vi "Node - Read Local Table.vi"(8 "error in (no error)":errorcluster, 10 "Node Name":string, 11 "Compiled.Settings In":T1) -> (0 "error out":errorcluster, 2 "Local Channels Table out":string[][](array[string]), 3 "Compiled.Settings Out":T1)   [LabVIEW 2016, in "PXImc Custom Device System Explorer.lvlib"]
uses:
  PXImc Custom Device System Explorer.lvlib
  Shared/Compiled.Settings.ctl
  <vilib>/NI Veristand/VeriStand Data/Byte Buffer/Byte Buffer.lvclass
  PXImc Router/Controls/Target Type.ctl
  PXImc Router/Controls/Router - Configuration.ctl
  PXImc Router/Controls/Router/Node Block R-W Properties.ctl
  PXImc Router/Controls/Router/Block Properties.ctl
  PXImc Router/Controls/Router/Router - PXImc Properties.ctl
  PXImc Router/Controls/Router/Router - PXImc Card Properties.ctl
  PXImc Router/Controls/Node Data.ctl
  PXImc Router/Controls/Node/Node - PXImc Parameters.ctl
  PXImc Router/Controls/Node/Node - Writer Data.ctl
  PXImc Router/Controls/Node/Node Ch Properties.ctl
  PXImc Router/Controls/Data Type.ctl
  PXImc Router/Controls/Node/Node - Readers Data.ctl
  PXImc Router/Controls/Node/Node - Reader Data.ctl
  <vilib>/Utility/file.llb/Read Delimited Spreadsheet (string).vi
  PXImc Router/PXImc Router.lvlib
  Shared/PXImc Custom Device Shared.lvlib
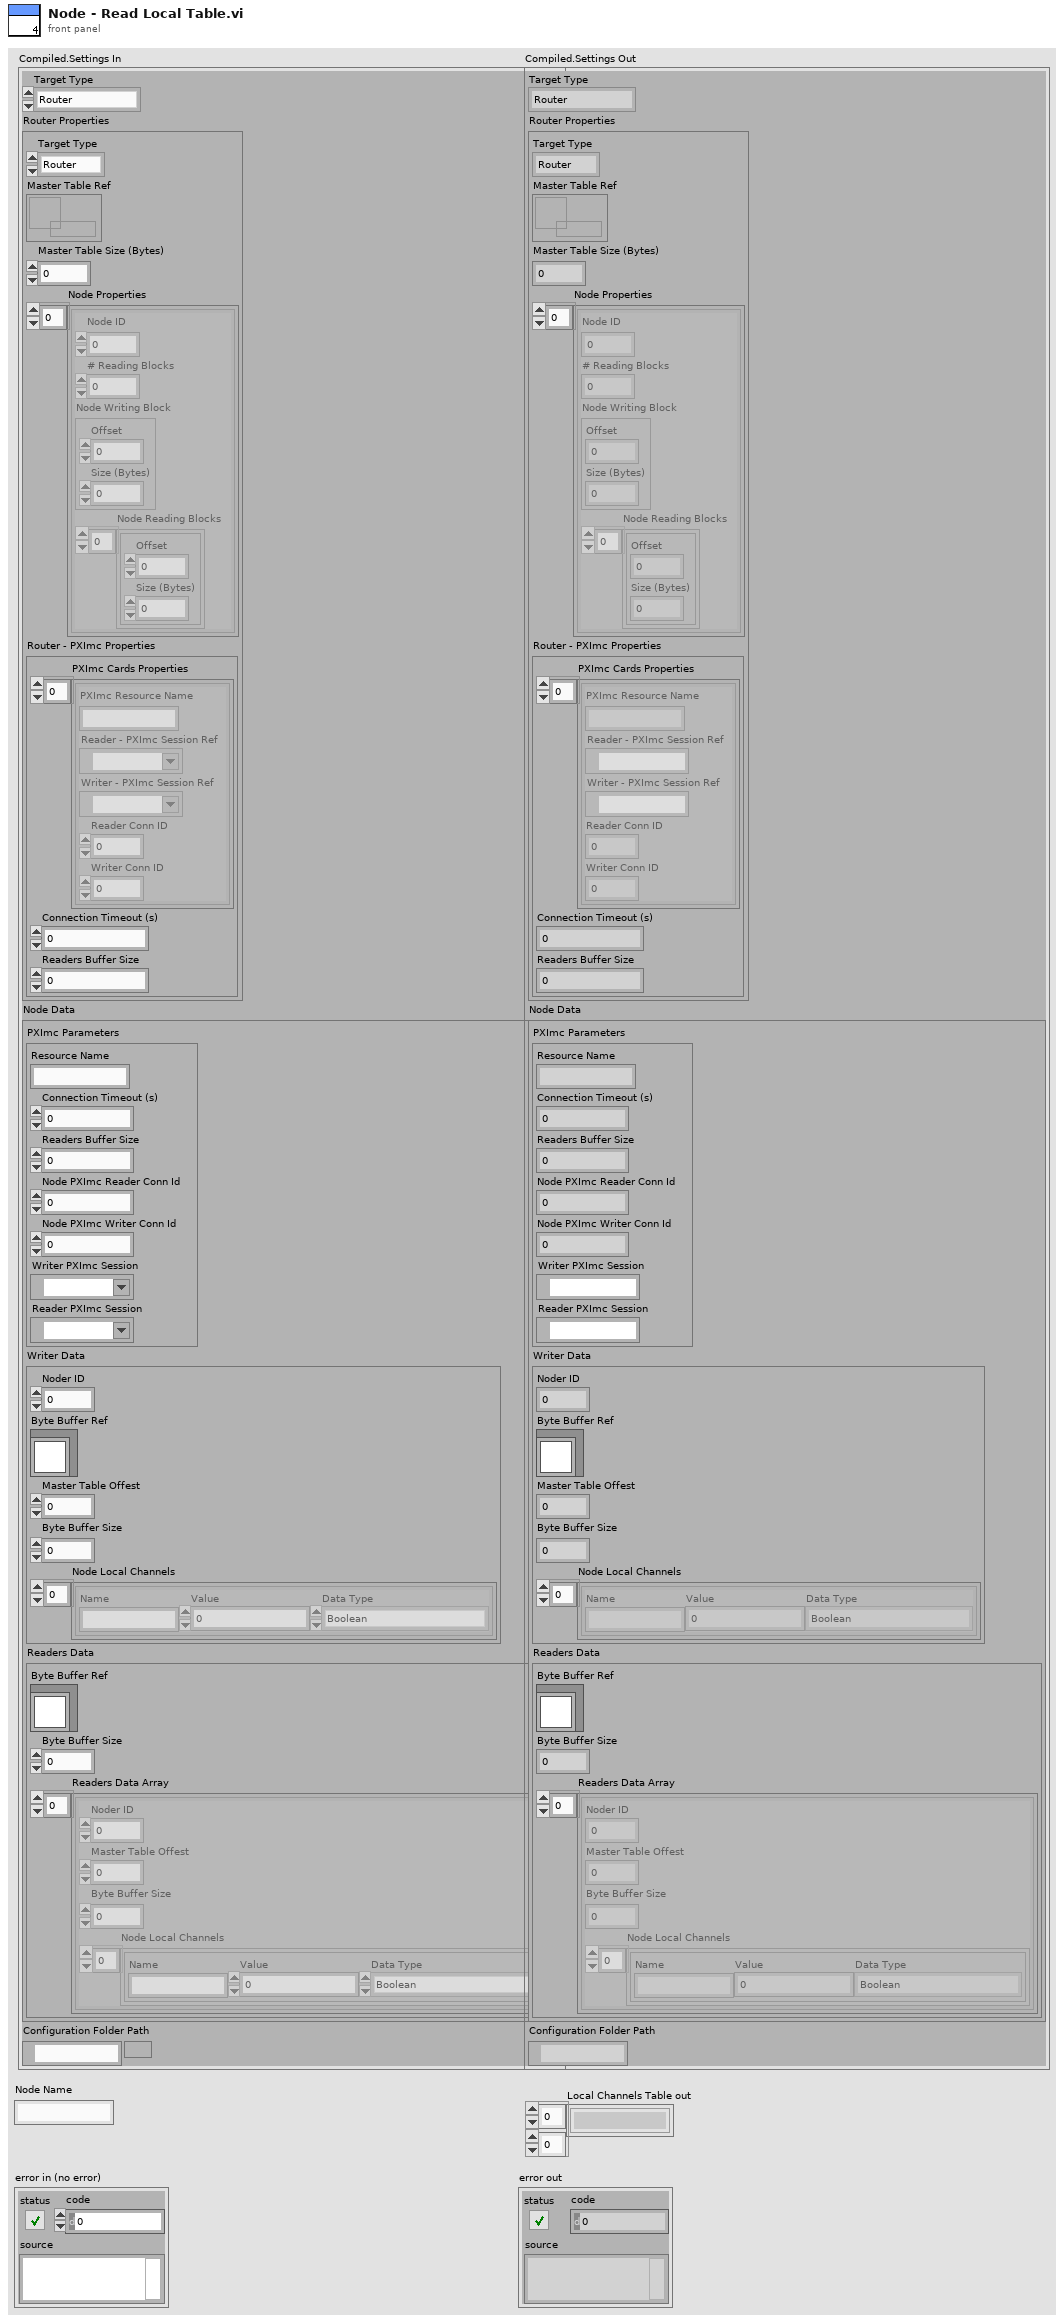
[diagram p1: front panel]
types:
  T1 = typedef "PXImc Custom Device Shared.lvlib/Compiled.Settings.ctl" = cluster{"Target Type":T2, "Router Properties":T3, "Node Data":T8, "Configuration Folder Path":path}
  T2 = typedef "PXImc Router.lvlib/Target Type.ctl" = enum16{"Router", "Node"}
  T3 = typedef "PXImc Router.lvlib/Router - Configuration.ctl" = cluster{"Target Type":T2, "Master Table Ref":refnum<data-value>, "Master Table Size (Bytes)":u32, "Node Properties":T4[], "Router - PXImc Properties":T6}
  T4 = typedef "PXImc Router.lvlib/Node Block R-W Properties.ctl" = cluster{"Node ID":u32, "# Reading Blocks":u32, "Node Writing Block":T5, "Node Reading Blocks":T5[]}
  T5 = typedef "PXImc Router.lvlib/Block Properties.ctl" = cluster{"Offset":u32, "Size (Bytes)":u32}
  T6 = typedef "PXImc Router.lvlib/Router - PXImc Properties.ctl" = cluster{"PXImc Cards Properties":T7[], "Connection Timeout (s)":dbl, "Readers Buffer Size":u64}
  T7 = typedef "PXImc Router.lvlib/Router - PXImc Card Properties.ctl" = cluster{"PXImc Resource Name":string, "Reader - PXImc Session Ref":refnum<k21>, "Writer - PXImc Session Ref":refnum<k21>, "Reader Conn ID":u16, "Writer Conn ID":u16}
  T8 = typedef "PXImc Router.lvlib/Node Data.ctl" = cluster{"PXImc Parameters":T9, "Writer Data":T10, "Readers Data":T13}
  T9 = typedef "PXImc Router.lvlib/Node - PXImc Parameters.ctl" = cluster{"Resource Name":string, "Connection Timeout (s)":dbl, "Readers Buffer Size":u64, "Node PXImc Reader Conn Id":u16, "Node PXImc Writer Conn Id":u16, "Writer PXImc Session":refnum<k21>, "Reader PXImc Session":refnum<k21>}
  T10 = typedef "PXImc Router.lvlib/Node - Writer Data.ctl" = cluster{"Noder ID":u32, "Byte Buffer Ref":refnum<class "Byte Buffer.lvclass">, "Master Table Offest":u32, "Byte Buffer Size":u32, "Node Local Channels":T11[]}
  T11 = typedef "PXImc Router.lvlib/Node Ch Properties.ctl" = cluster{"Name":string, "Value":dbl, "Data Type":T12}
  T12 = typedef "PXImc Router.lvlib/Data Type.ctl" = enum16{"Boolean", "SGL", "DBL", "I8", "I16", "I32", "I64", "U8", "U16", "U32", "U64"}
  T13 = typedef "PXImc Router.lvlib/Node - Readers Data.ctl" = cluster{"Byte Buffer Ref":refnum<class "Byte Buffer.lvclass">, "Byte Buffer Size":u64, "Readers Data Array":T14[]}
  T14 = typedef "PXImc Router.lvlib/Node - Reader Data.ctl" = cluster{"Noder ID":u32, "Master Table Offest":u32, "Byte Buffer Size":u64, "Node Local Channels":T11[]}
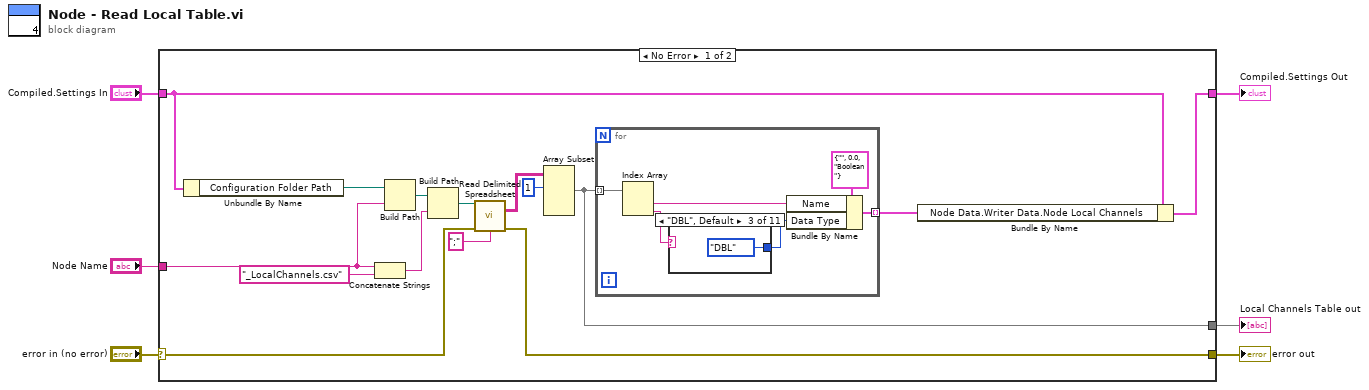
[diagram p0: block diagram]
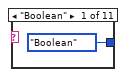
[diagram p2: hidden frame]
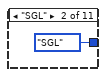
[diagram p3: hidden frame]
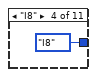
[diagram p4: hidden frame]
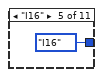
[diagram p5: hidden frame]
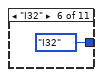
[diagram p6: hidden frame]
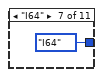
[diagram p7: hidden frame]
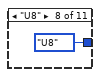
[diagram p8: hidden frame]
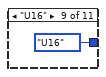
[diagram p9: hidden frame]
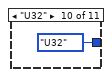
[diagram p10: hidden frame]
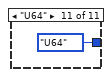
[diagram p11: hidden frame]
diagram:
  n1 = case shown="No Error" "error in (no error)" {
    selector: "error in (no error)" -> [w9 w39]
    tunnel: "Compiled.Settings In" -> [w17 w40]
    tunnel: [w18 w40] -> w5
    tunnel: [w8 w39] -> w3
    tunnel: "Node Name" -> [w15 _]
    tunnel: [w7 _] -> w1
    frame No Error {
      n2 = Unbundle By Name(w17) -> ("Configuration Folder Path"=w16:path)
      n3 = Concatenate Strings(w15, "_LocalChannels.csv" ("name or relative path")) -> (w13:string)
      n4 = Build Path(base path=w16, name or relative path=w15) -> (appended path=w21:path)
      n5 = Build Path(base path=w21, name or relative path=w13) -> (appended path=w20:path)
      n6 = call-poly <vilib>:"Read Delimited Spreadsheet.vi"("file path (dialog if empty)"=w20, "error in (no error)"=w9, "delimiter (\\t)"=";" ("delimiter (\\t)")) -> ("all rows"=w12:string[][], "error out"=w8:errorcluster)  [unwired: 7 in, 4 out]
      n7 = Array Subset(array=w12, index (row)=1 ("index")) -> (w7:string[][])  [unwired: 3 in]
      n8 = for {
        tunnel: [w27] -> w10 mode=indexing
        tunnel: w7 -> [w26] mode=indexing
        n9 = Index Array(array=w26) -> (element #1=w23:string, element #2=w22:string)  [unwired: 2 in]
        n10 = case shown="\"DBL\", Default" w22 {
          tunnel: [Data_Type."Boolean" ("Data Type") Data_Type."SGL" ("Data Type") Data_Type."DBL" ("Data Type") Data_Type."I8" ("Data Type") Data_Type."I16" ("Data Type") Data_Type."I32" ("Data Type") Data_Type."I64" ("Data Type") Data_Type."U8" ("Data Type") Data_Type."U16" ("Data Type") Data_Type."U32" ("Data Type") Data_Type."U64" ("Data Type")] -> w25
          frame "Boolean" {
          }
          frame "SGL" {
          }
          frame "DBL", Default {
          }
          frame "I8" {
          }
          frame "I16" {
          }
          frame "I32" {
          }
          frame "I64" {
          }
          frame "U8" {
          }
          frame "U16" {
          }
          frame "U32" {
          }
          frame "U64" {
          }
        }
        n11 = Bundle By Name(cluster=T11 {"Name"="", "Value"=0.0, "Data Type"=enum."Boolean"} ("Node Ch Properties"), "Name"=w23, "Data Type"=w25) -> (w27:T11)
      }
      n12 = Bundle By Name(cluster=w17, "Node Data.Writer Data.Node Local Channels"=w10) -> (w18:T1)
    }
    frame Error {
    }
  }
  "Compiled.Settings Out" <- w5
  "error out" <- w3
  "Local Channels Table out" <- w1
